vi "CIFTag Update Test Cases.vi"() -> (0 "error out":errorcluster, 2 "status":string, 3 "pass":bool)   [LabVIEW 2021]
uses:
  Double/CIFTagDouble.lvclass
  CIFChannels/Typedef/Direction.ctl
  CIFChannels/CIFChannels.lvclass
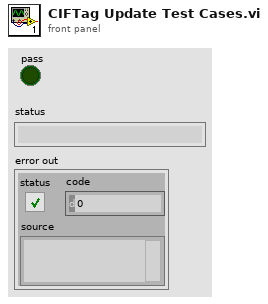
[diagram p1: front panel]
types:
  T1 = typedef "CIFChannels.lvclass/Direction.ctl" = enum16{"Publisher", "Subscriber"}
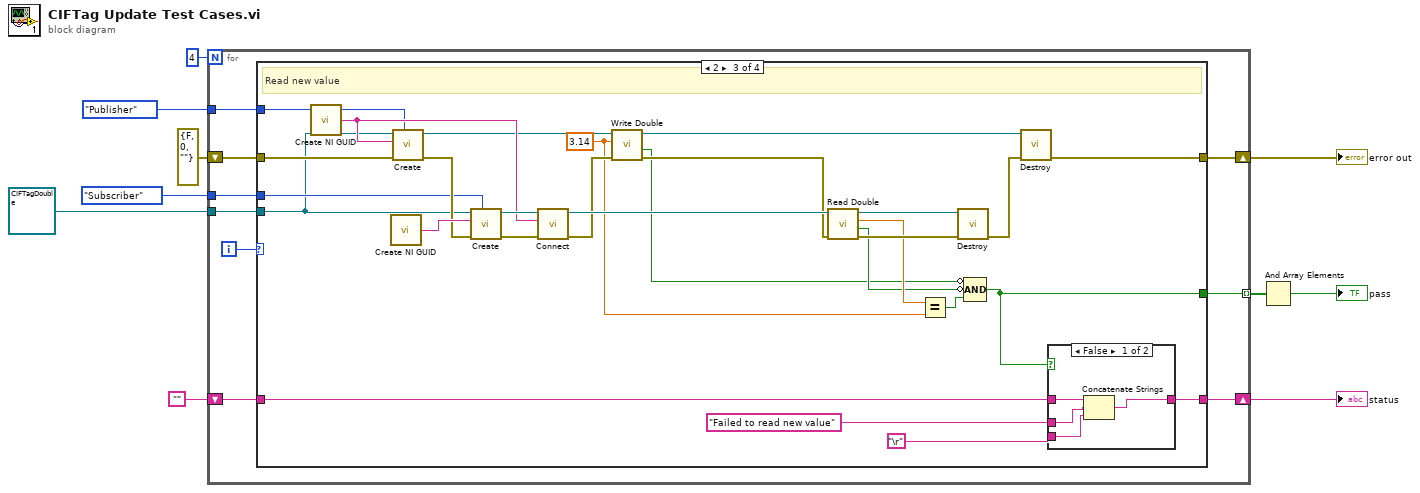
[diagram p0: block diagram]
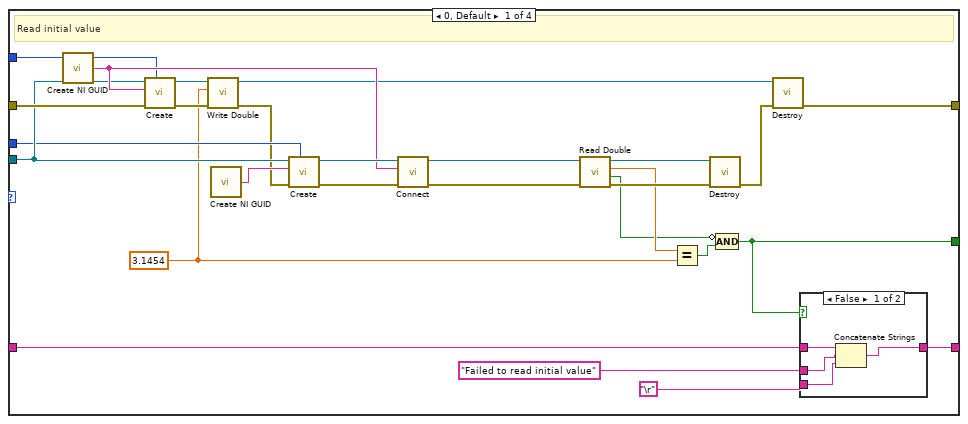
[diagram p2: hidden frame]
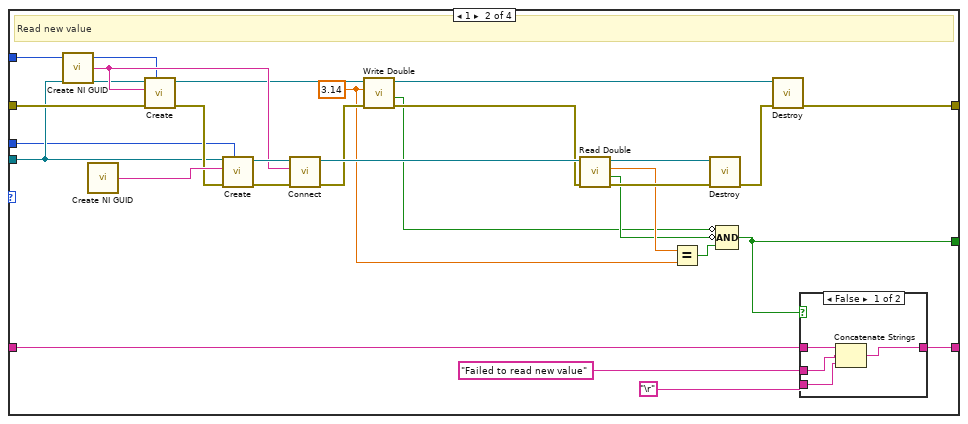
[diagram p4: hidden frame]
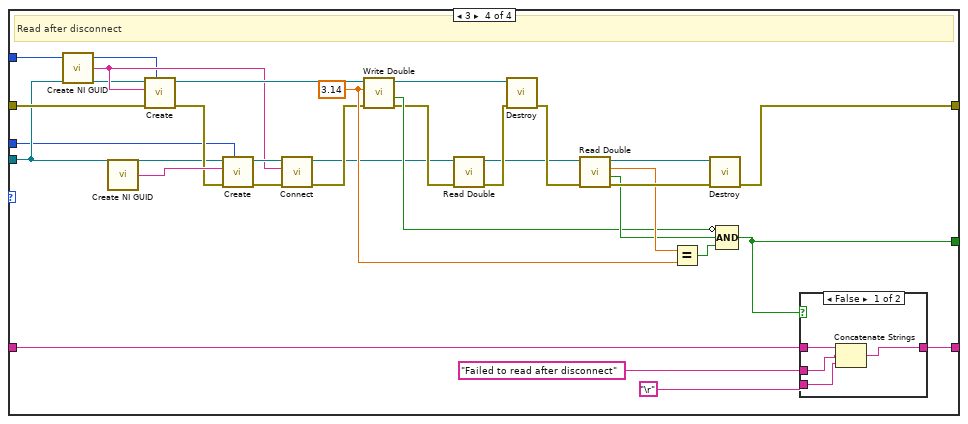
[diagram p7: hidden frame]
diagram:
  n1 = for {
    N: 4 -> [_]
    tunnel: [w19] -> w10 mode=indexing
    shift-right: [w17] -> w5
    shift-left: errorcluster {"status"=FALSE, "code"=0, "source"=""} ("error out") -> [w18]
    shift-right: [w14] -> w6
    shift-left: "" -> [w15]
    tunnel: refnum<class "CIFTagDouble.lvclass"> refnum ("CIFTagDouble.lvclass") -> [w13]
    tunnel: Direction."Publisher" ("Direction") -> [w12]
    tunnel: Direction."Subscriber" ("Direction") -> [w11]
    i -> [w16]
    n2 = case shown="2" w16 {
      tunnel: [w29 w62 w95 w136] -> w19
      tunnel: w18 -> [w42 w75 w108 w143]
      tunnel: [w32 w65 w98 w127] -> w17
      tunnel: w15 -> [w46 w79 w112 w147]
      tunnel: [w45 w78 w111 w146] -> w14
      tunnel: w13 -> [w26 w54 w85 w120]
      tunnel: w12 -> [w27 w53 w87 w119]
      tunnel: w11 -> [w25 w52 w86 w118]
      frame 0, Default {
        w20 = 3.1454
        # "Read initial value"
        n3 = call <vilib>:"Create NI GUID.vi"() -> ("NI GUID"=w38:string)
        n4 = call-dynamic "Create.vi"("Direction"=w27, "error in (no error)"=w42, "Name"=w38, "CIFTag in"=w26) -> ("error out"=w23:errorcluster, "CIFTag out"=w24:refnum<class "CIFTagDouble.lvclass">)  [unwired: 6 in]
        n5 = call-dynamic "Write Double.vi"("error in (no error)"=w23, "Data"=w20, "CIFTag in"=w24) -> ("error out"=w21:errorcluster, "CIFTag out"=w22:refnum<class "CIFTagDouble.lvclass">)  [unwired: 6 in, 1 out]
        n6 = call <vilib>:"Create NI GUID.vi"() -> ("NI GUID"=w41:string)
        n7 = call-dynamic "Create.vi"("Direction"=w25, "error in (no error)"=w21, "Name"=w41, "CIFTag in"=w26) -> ("error out"=w39:errorcluster, "CIFTag out"=w40:refnum<class "CIFTagDouble.lvclass">)  [unwired: 6 in]
        n8 = call-dynamic "Connect.vi"("error in (no error)"=w39, "Connection Name"=w38, "CIFTag in"=w40) -> ("error out"=w36:errorcluster, "CIFTag out"=w37:refnum<class "CIFTagDouble.lvclass">)  [unwired: 7 in]
        n9 = call-dynamic "Read Double.vi"("error in (no error)"=w36, "CIFTag in"=w37) -> ("error out"=w34:errorcluster, "timed out?"=w28:bool, "Data"=w31:dbl, "CIFTag out"=w35:refnum<class "CIFTagDouble.lvclass">)  [unwired: 6 in]
        n10 = Equal?(x=w31, y=w20) -> (x = y?=w30:bool)
        n11 = call-dynamic "Destroy.vi"("error in (no error)"=w34, "CIFTag in"=w35) -> ("error out"=w33:errorcluster)  [unwired: 8 in, 1 out]
        n12 = Compound Arithmetic op=AND(invert w28, w30) -> (w29:bool)
        n13 = call-dynamic "Destroy.vi"("error in (no error)"=w33, "CIFTag in"=w22) -> ("error out"=w32:errorcluster)  [unwired: 8 in, 1 out]
        n14 = case shown="False" w29 {
          tunnel: w46 -> [w50 w51]
          tunnel: [w47 w51] -> w45
          tunnel: "Failed to read initial value" -> [w49 _]
          tunnel: "\r" -> [w48 _]
          frame False {
            n15 = Concatenate Strings(w50, w49, w48) -> (w47:string)
          }
          frame True {
          }
        }
      }
      frame 1 {
        w55 = 3.14 ("Data")
        # "Read new value"
        n16 = call <vilib>:"Create NI GUID.vi"() -> ("NI GUID"=w70:string)
        n17 = call <vilib>:"Create NI GUID.vi"() -> ("NI GUID"=w74:string)
        n18 = call-dynamic "Create.vi"("Direction"=w53, "error in (no error)"=w75, "Name"=w70, "CIFTag in"=w54) -> ("error out"=w73:errorcluster, "CIFTag out"=w60:refnum<class "CIFTagDouble.lvclass">)  [unwired: 6 in]
        n19 = call-dynamic "Create.vi"("Direction"=w52, "error in (no error)"=w73, "Name"=w74, "CIFTag in"=w54) -> ("error out"=w71:errorcluster, "CIFTag out"=w72:refnum<class "CIFTagDouble.lvclass">)  [unwired: 6 in]
        n20 = call-dynamic "Connect.vi"("error in (no error)"=w71, "Connection Name"=w70, "CIFTag in"=w72) -> ("error out"=w59:errorcluster, "CIFTag out"=w69:refnum<class "CIFTagDouble.lvclass">)  [unwired: 7 in]
        n21 = call-dynamic "Write Double.vi"("error in (no error)"=w59, "Data"=w55, "CIFTag in"=w60) -> ("error out"=w58:errorcluster, "timed out?"=w56:bool, "CIFTag out"=w57:refnum<class "CIFTagDouble.lvclass">)  [unwired: 6 in]
        n22 = call-dynamic "Read Double.vi"("error in (no error)"=w58, "CIFTag in"=w69) -> ("error out"=w67:errorcluster, "timed out?"=w61:bool, "Data"=w64:dbl, "CIFTag out"=w68:refnum<class "CIFTagDouble.lvclass">)  [unwired: 6 in]
        n23 = Equal?(x=w64, y=w55) -> (x = y?=w63:bool)
        n24 = call-dynamic "Destroy.vi"("error in (no error)"=w67, "CIFTag in"=w68) -> ("error out"=w66:errorcluster)  [unwired: 8 in, 1 out]
        n25 = Compound Arithmetic op=AND(invert w56, invert w61, w63) -> (w62:bool)
        n26 = call-dynamic "Destroy.vi"("error in (no error)"=w66, "CIFTag in"=w57) -> ("error out"=w65:errorcluster)  [unwired: 8 in, 1 out]
        n27 = case shown="False" w62 {
          tunnel: w79 -> [w83 w84]
          tunnel: [w80 w84] -> w78
          tunnel: "Failed to read new value" -> [w82 _]
          tunnel: "\r" -> [w81 _]
          frame False {
            n28 = Concatenate Strings(w83, w82, w81) -> (w80:string)
          }
          frame True {
          }
        }
      }
      frame 2 {
        w88 = 3.14 ("Data")
        # "Read new value"
        n29 = call <vilib>:"Create NI GUID.vi"() -> ("NI GUID"=w103:string)
        n30 = call <vilib>:"Create NI GUID.vi"() -> ("NI GUID"=w107:string)
        n31 = call-dynamic "Create.vi"("Direction"=w87, "error in (no error)"=w108, "Name"=w103, "CIFTag in"=w85) -> ("error out"=w106:errorcluster, "CIFTag out"=w93:refnum<class "CIFTagDouble.lvclass">)  [unwired: 6 in]
        n32 = call-dynamic "Create.vi"("Direction"=w86, "error in (no error)"=w106, "Name"=w107, "CIFTag in"=w85) -> ("error out"=w104:errorcluster, "CIFTag out"=w105:refnum<class "CIFTagDouble.lvclass">)  [unwired: 6 in]
        n33 = call-dynamic "Connect.vi"("error in (no error)"=w104, "Connection Name"=w103, "CIFTag in"=w105) -> ("error out"=w92:errorcluster, "CIFTag out"=w102:refnum<class "CIFTagDouble.lvclass">)  [unwired: 7 in]
        n34 = call-dynamic "Write Double.vi"("error in (no error)"=w92, "Data"=w88, "CIFTag in"=w93) -> ("error out"=w91:errorcluster, "timed out?"=w89:bool, "CIFTag out"=w90:refnum<class "CIFTagDouble.lvclass">)  [unwired: 6 in]
        n35 = call-dynamic "Read Double.vi"("error in (no error)"=w91, "CIFTag in"=w102) -> ("error out"=w100:errorcluster, "timed out?"=w94:bool, "Data"=w97:dbl, "CIFTag out"=w101:refnum<class "CIFTagDouble.lvclass">)  [unwired: 6 in]
        n36 = Equal?(x=w97, y=w88) -> (x = y?=w96:bool)
        n37 = call-dynamic "Destroy.vi"("error in (no error)"=w100, "CIFTag in"=w101) -> ("error out"=w99:errorcluster)  [unwired: 8 in, 1 out]
        n38 = Compound Arithmetic op=AND(invert w89, invert w94, w96) -> (w95:bool)
        n39 = call-dynamic "Destroy.vi"("error in (no error)"=w99, "CIFTag in"=w90) -> ("error out"=w98:errorcluster)  [unwired: 8 in, 1 out]
        n40 = case shown="False" w95 {
          tunnel: w112 -> [w116 w117]
          tunnel: [w113 w117] -> w111
          tunnel: "Failed to read new value" -> [w115 _]
          tunnel: "\r" -> [w114 _]
          frame False {
            n41 = Concatenate Strings(w116, w115, w114) -> (w113:string)
          }
          frame True {
          }
        }
      }
      frame 3 {
        w128 = 3.14 ("Data")
        # "Read after disconnect"
        n42 = call <vilib>:"Create NI GUID.vi"() -> ("NI GUID"=w121:string)
        n43 = call <vilib>:"Create NI GUID.vi"() -> ("NI GUID"=w142:string)
        n44 = call-dynamic "Create.vi"("Direction"=w119, "error in (no error)"=w143, "Name"=w121, "CIFTag in"=w120) -> ("error out"=w141:errorcluster, "CIFTag out"=w134:refnum<class "CIFTagDouble.lvclass">)  [unwired: 6 in]
        n45 = call-dynamic "Create.vi"("Direction"=w118, "error in (no error)"=w141, "Name"=w142, "CIFTag in"=w120) -> ("error out"=w124:errorcluster, "CIFTag out"=w125:refnum<class "CIFTagDouble.lvclass">)  [unwired: 6 in]
        n46 = call-dynamic "Connect.vi"("error in (no error)"=w124, "Connection Name"=w121, "CIFTag in"=w125) -> ("error out"=w123:errorcluster, "CIFTag out"=w122:refnum<class "CIFTagDouble.lvclass">)  [unwired: 7 in]
        n47 = call-dynamic "Write Double.vi"("error in (no error)"=w123, "Data"=w128, "CIFTag in"=w134) -> ("error out"=w132:errorcluster, "timed out?"=w133:bool, "CIFTag out"=w131:refnum<class "CIFTagDouble.lvclass">)  [unwired: 6 in]
        n48 = call-dynamic "Read Double.vi"("error in (no error)"=w132, "CIFTag in"=w122) -> ("error out"=w130:errorcluster, "CIFTag out"=w126:refnum<class "CIFTagDouble.lvclass">)  [unwired: 6 in, 2 out]
        n49 = call-dynamic "Destroy.vi"("error in (no error)"=w130, "CIFTag in"=w131) -> ("error out"=w129:errorcluster)  [unwired: 8 in, 1 out]
        n50 = call-dynamic "Read Double.vi"("error in (no error)"=w129, "CIFTag in"=w126) -> ("error out"=w139:errorcluster, "timed out?"=w135:bool, "Data"=w138:dbl, "CIFTag out"=w140:refnum<class "CIFTagDouble.lvclass">)  [unwired: 6 in]
        n51 = Equal?(x=w138, y=w128) -> (x = y?=w137:bool)
        n52 = call-dynamic "Destroy.vi"("error in (no error)"=w139, "CIFTag in"=w140) -> ("error out"=w127:errorcluster)  [unwired: 8 in, 1 out]
        n53 = Compound Arithmetic op=AND(invert w133, w135, w137) -> (w136:bool)
        n54 = case shown="False" w136 {
          tunnel: w147 -> [w151 w152]
          tunnel: [w148 w152] -> w146
          tunnel: "Failed to read after disconnect" -> [w150 _]
          tunnel: "\r" -> [w149 _]
          frame False {
            n55 = Concatenate Strings(w151, w150, w149) -> (w148:string)
          }
          frame True {
          }
        }
      }
    }
  }
  "error out" <- w5
  "status" <- w6
  n56 = And Array Elements(Boolean array=w10) -> (logical AND=→"pass":bool)
